vi "Read Number1.vi"(8 "error in (no error)":errorcluster, 11 "Numbers in":refnum<class "Numbers.lvclass">) -> (0 "error out":errorcluster, 2 "Number1":dbl, 3 "Numbers out":refnum<class "Numbers.lvclass">)   [LabVIEW 2017, in "Numbers.lvclass"]
uses:
  Numbers.lvclass
  Numbers.lvclass/Numbers.ctl
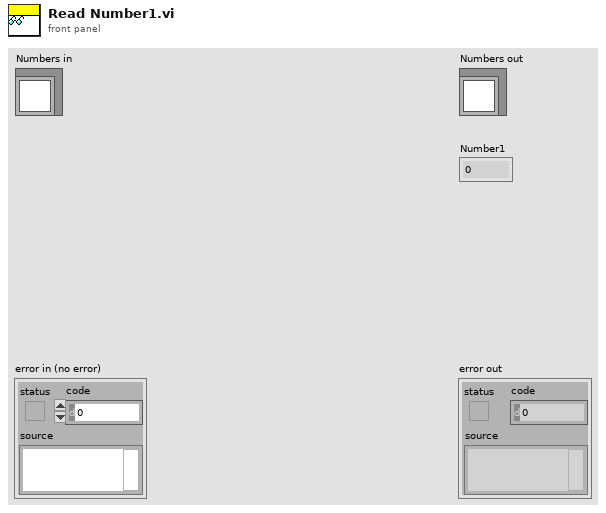
[diagram p1: front panel]
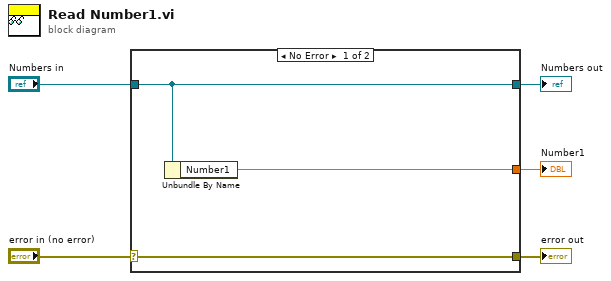
[diagram p0: block diagram]
diagram:
  n1 = case shown="No Error" "error in (no error)" {
    selector: "error in (no error)" -> [w8 w9]
    tunnel: [w8 w9] -> w4
    tunnel: [w7 w10] -> w2
    tunnel: "Numbers in" -> [w7 w10]
    tunnel: [w6 _] -> w1
    frame No Error {
      n2 = Unbundle By Name(w7) -> ("Number1"=w6:dbl)
    }
    frame Error {
    }
  }
  "error out" <- w4
  "Numbers out" <- w2
  "Number1" <- w1
